vi "FlatToRichProtocol_Request.vi"(5 "OutputClusterType":T1, 11 "InputCluster":T2) -> (3 "OutputCluster":T1)   [LabVIEW 2021, in "Unary_client.lvlib"]
uses:
  Unary_client.lvlib
  Protocol_Request_Flat.ctl
  Protocol_Request.ctl
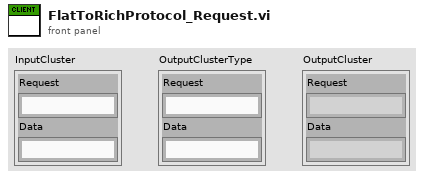
[diagram p1: front panel]
types:
  T1 = typedef "Unary_client.lvlib/Protocol_Request.ctl" = cluster{"Request":string, "Data":string}
  T2 = typedef "Unary_client.lvlib/Protocol_Request_Flat.ctl" = cluster{"Request":string, "Data":string}
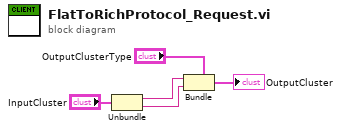
[diagram p0: block diagram]
diagram:
  n1 = Unbundle "Unbundle"("InputCluster") -> ("Request"=w2:string, "Data"=w1:string)
  n2 = Bundle "Bundle"(cluster="OutputClusterType", "Request"=w2, "Data"=w1) -> (→"OutputCluster":T1)
